vi "DLL_version.vi"(0 "USBTransferNfoPtr":u32, 11 "error in (no error)":errorcluster) -> (4 "USBTransferNfoPtr out":u32, 6 "DLL version":string="1.00", 15 "error out":errorcluster)   [LabVIEW 2017, in "ZBOX_IS.lvlib"]
uses:
  ZBOX_IS.lvlib
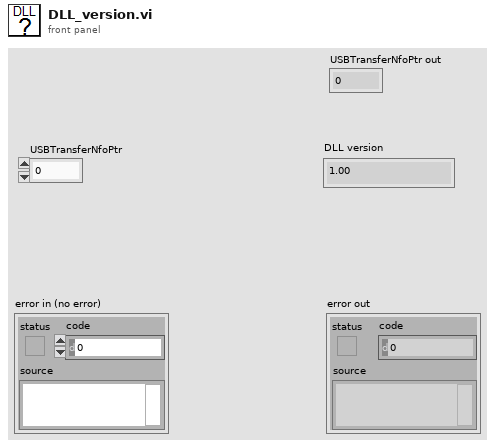
[diagram p1: front panel]
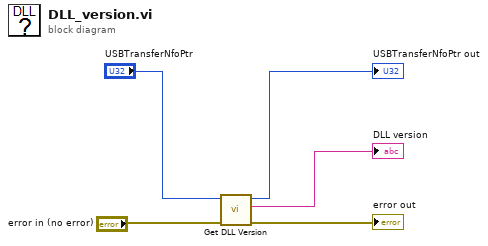
[diagram p0: block diagram]
diagram:
  n1 = call "Get DLL Version.vi"("error in (no error)"="error in (no error)", "USBTransferNfoPtr"="USBTransferNfoPtr") -> ("error out"=→"error out":errorcluster, "function return"=→"DLL version":string, "USBTransferNfoPtr out"=→"USBTransferNfoPtr out":u32)  [unwired: 7 in]
